vi "dump.vi"(8 "error in (no error)":errorcluster, 10 "indent":T1, 11 "Node in":refnum<class "Node.lvclass">) -> (0 "error out":errorcluster, 2 "mlir":string, 3 "Node out":refnum<class "Node.lvclass">)   [LabVIEW 2020, in "mlir.lvlib" / "Node.lvclass"]
uses:
  Node.lvclass
  indent.ctl
  Node.lvclass/Node.ctl
  mlir.lvlib
panel:
  # "Dumps the AST node and its children in MLIR format."
  # "String representing the AST in MLIR."
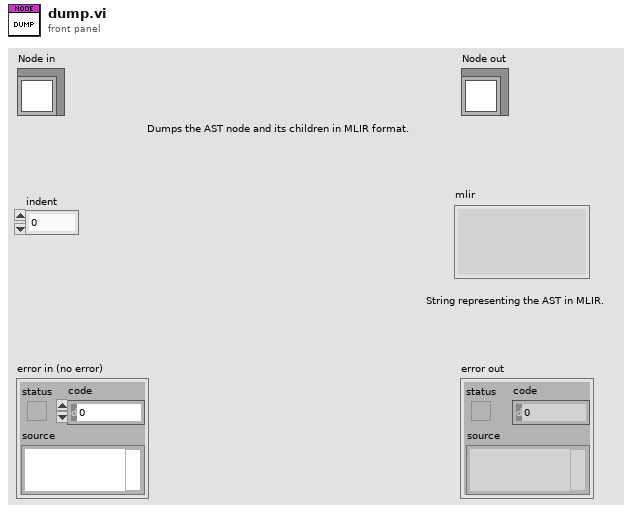
[diagram p1: front panel]
types:
  T1 = typedef "mlir.lvlib/indent.ctl" = u32
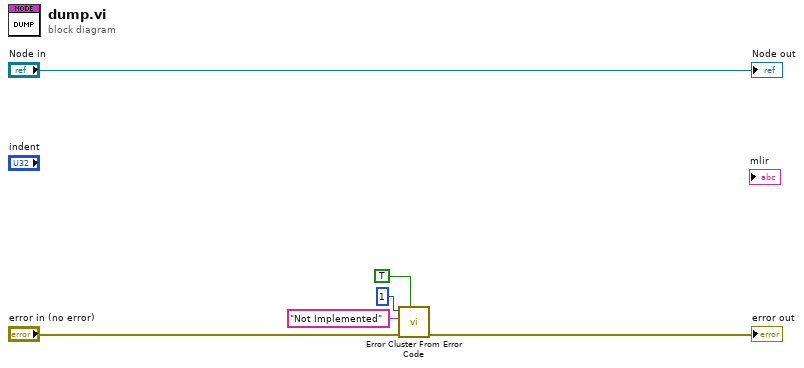
[diagram p0: block diagram]
diagram:
  n1 = call <vilib>:"Error Cluster From Error Code.vi"("show call chain? (False)"=TRUE, "error in (no error)"="error in (no error)", "error message (\"\")"="Not Implemented" ("error message (\"\")"), "error code (0)"=1) -> ("error out"=→"error out":errorcluster)  [unwired: 5 in]
  "Node out" <- "Node in"
